vi "DB Module.vi"(6 "connection information":path, 8 "error in (no error)":errorcluster, 11 "Mode (Get Connection)":T2=enum."Get Connection") -> (0 "error out":errorcluster, 3 "connection reference":T1)   [LabVIEW 2012, in "Database Lib.lvlib"]
doc: "A reentrant functional global. Holds a connection to a database and the udl file associated with the database. Will reconnect to the database if the connection is lost.\n\nModes: Open Connection, Get Connection, Close Connection"
uses:
  Database Lib.lvlib
  DB Connection Mode enum.ctl
  Utility/database/Connection.llb/Conn ObjectReference.ctl
  Utility/database/Connection.llb/Conn Get Properties.vi
  Utility/database/NI_Database_API_64.lvlib
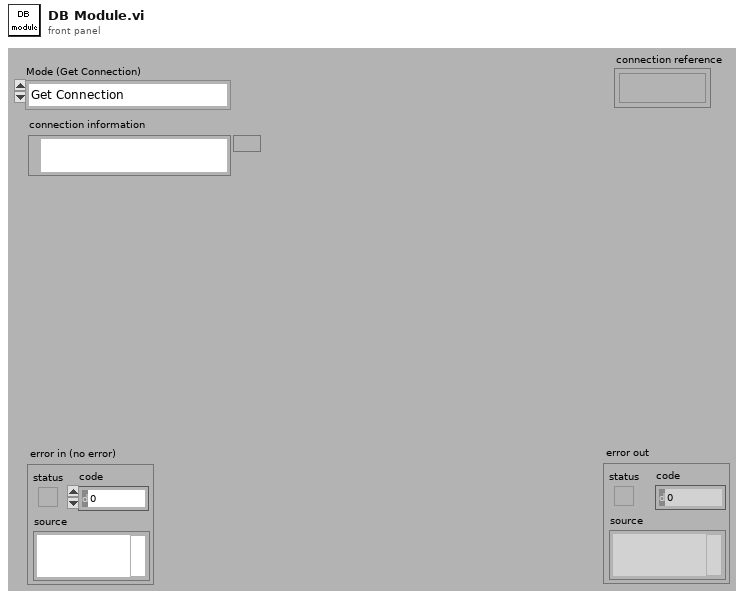
[diagram p1: front panel]
types:
  T1 = typedef "NI_Database_API_64.lvlib/Conn ObjectReference.ctl" = refnum<k1>
  T2 = typedef "Database Lib.lvlib/DB Connection Mode enum.ctl" = enum16{"Connect", "Get Connection", "Disconnect"}
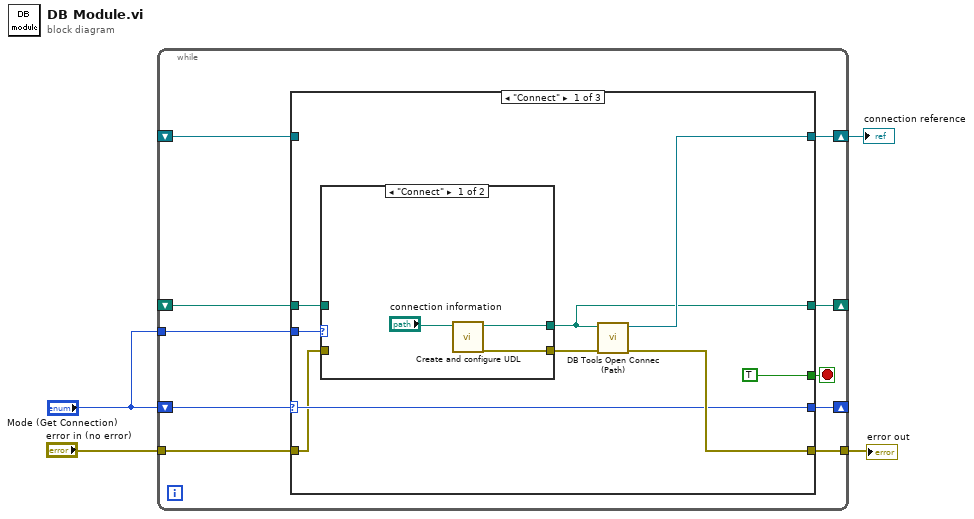
[diagram p0: block diagram]
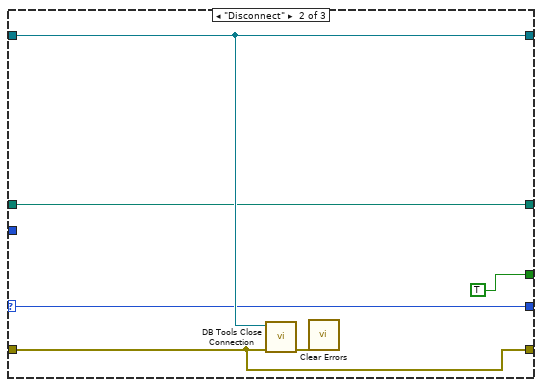
[diagram p3: hidden frame]
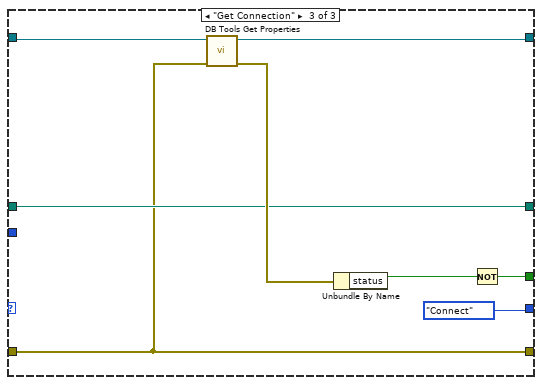
[diagram p4: hidden frame]
diagram:
  n1 = while {
    tunnel: [w13] -> w4
    tunnel: "error in (no error)" -> [w12]
    shift-right: [w11] -> w2
    shift-left: _ -> [w10]
    shift-right: [w8] -> _
    shift-left: "Mode (Get Connection)" -> [w14]
    tunnel: "Mode (Get Connection)" -> [w7]
    shift-right: [w6] -> _
    shift-left: _ -> [w5]
    stop <- w9 stop-if-true
    n2 = case shown="\"Connect\"" w14 {
      selector: w14 -> [w20 w32 _]
      tunnel: [w23 w30 w35] -> w13
      tunnel: [w22 w34 w41] -> w11
      tunnel: w12 -> [w15 w30 w35]
      tunnel: w10 -> [_ w34 w42]
      tunnel: [TRUE TRUE w39] -> w9
      tunnel: [w20 w32 DB_Connection_Mode_enum."Connect" ("Mode")] -> w8
      tunnel: w7 -> [w19 _ _]
      tunnel: [w17 w31 w36] -> w6
      tunnel: w5 -> [w18 w31 w36]
      frame "Connect" {
        n3 = case shown="\"Connect\"" w19 {
          tunnel: [w25 w28] -> w17
          tunnel: w18 -> [_ w28]
          tunnel: [w24 w27] -> w16
          tunnel: w15 -> [_ w27]
          frame "Connect" {
            n4 = call "Create and configure UDL.vi"("file path (use dialog)"="connection information") -> ("error out"=w24:errorcluster, "UDL path"=w25:path)  [unwired: 1 in, 8 out]
          }
          frame "Get Connection", Default {
          }
        }
        n5 = call "DB Tools Open Connec (Path).vi"("error in (no error)"=w16, "connection information"=w17) -> ("error out"=w23:errorcluster, "connection reference"=w22:T1)  [unwired: 3 in, 3 out]
      }
      frame "Disconnect" {
        n6 = call "DB Tools Close Connection.vi"("error in (no error)"=w30, "connection reference"=w34) -> ("error out"=w29:errorcluster)  [unwired: 5 out]
        n7 = call <vilib>:"Clear Errors.vi"("error in (no error)"=w29) -> ()  [unwired: 7 out]
      }
      frame "Get Connection" {
        n8 = call-poly "DB Tools Get Properties.vi"("error in (no error)"=w35, "connection reference"=w42) -> ("error out"=w40:errorcluster, "connection reference out"=w41:T1)  [unwired: 4 out]
        n9 = Unbundle By Name(w40) -> ("status"=w38:bool)
        n10 = Not(x=w38) -> (.not. x?=w39:bool)
      }
    }
  }
  "error out" <- w4
  "connection reference" <- w2
